vi "BLD_Analysis.vi"() -> ()   [LabVIEW 2019]
uses:
  <vilib>/Analysis/5stat.llb/RMS (DBL).vi
  <vilib>/Analysis/baseanly.llb/Mean (DBL).vi
  <vilib>/express/express analysis/Spectral/Block/exnSpectralBlock spectral measurements power poly.vi
  <vilib>/express/express analysis/Spectral/Block/exnSpectralBlock spectral measurements power DDT.vi
  <vilib>/express/express analysis/Spectral/XNode/ExpressSpectralMeasurementsBlockNode.xnode
  <vilib>/Analysis/NI_AALBase.lvlib
  <vilib>/Analysis/NI_AALPro.lvlib
panel:
  in  "Sensitivity (V)":dbl=100000.0 format="%#_6p"
  in  "Tc (s)":i32=10000 format="%.0p"
  in  "Sampling Rate (Hz)":dbl=100000.0 format="%#_6p"
  in  "Samples (#)":i32=10000 format="%.0p"
  out "data":dynamicdata(graph) caption="APD Output"
  out "Photons/Pulse":ext=-1.22632021926945247725 format="%#.0g"
  in  "Repetition Rate (Hz)":ext[unit]=80000000.0 format="%#_6p"
  in  "Wavelength (m)":dbl=4e-07 format="%#_6p"
  out "Photons/Second":ext[unit]=-98105617.54155619818 format="%#.0p"
  out "Noise (W)":dbl=6.138754193845233e-11 format="%#.2p"
  out "Mean Power (W)":dbl=-4.8720373573303983e-11 format="%#.3p"
  in  "Gain (V/W)":dbl=2500000.0 format="%#_6p"
  in  "stop":bool
  out "Power Spectrum":dynamicdata(graph)=[{"t0"=timestamp(0 s since 1904-01-01), "dt"=1.0000000032596297, "Y"=array[25000 elements], "attributes"=variant("NI_ChannelName"=variant(string "Voltage (Power Spectrum)"), "NI_OriginalChannelName"=variant(string "Voltage"), "NI_UnitDescription"=variant(string "Volts"))}]
  # "Optical Input"
  # "APD"
  # "Lock-in"
  # "DAQ"
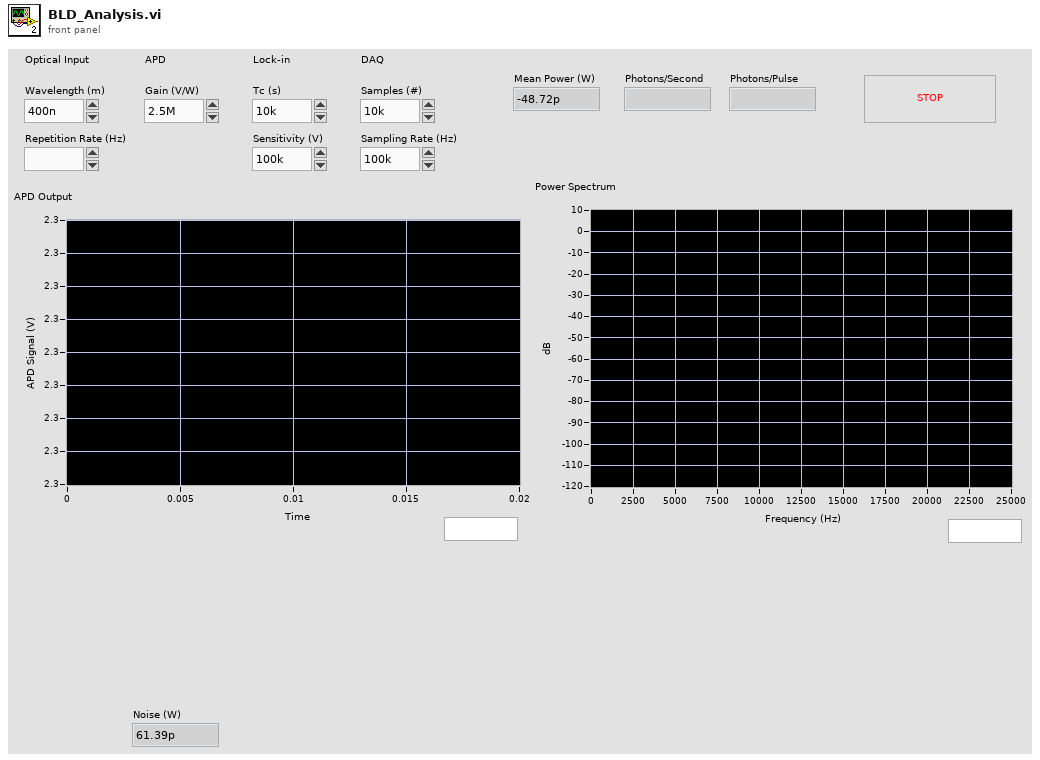
[diagram p1: front panel]
types:
  T1 = cluster{"averaging mode":u16, "weighting mode":u16, "number of averages":u32}
  T2 = cluster{"dB On (F)":bool, "unwrap phase (F)":bool, "convert to degree (F)":bool}
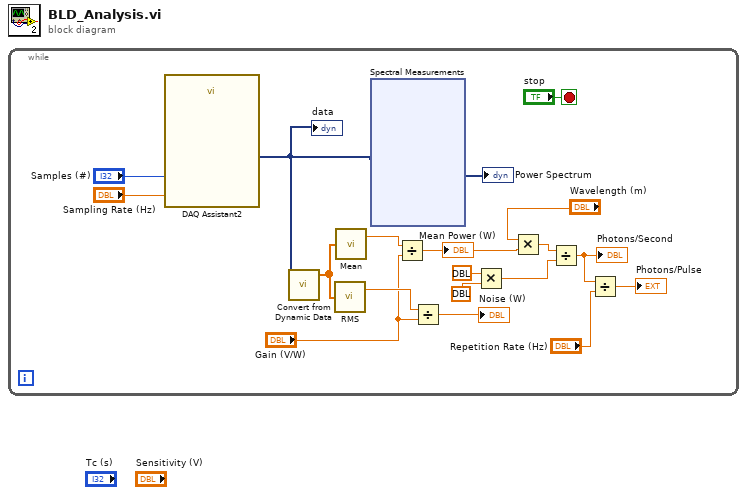
[diagram p0: block diagram]
diagram:
  n1 = while {
    stop <- "stop" stop-if-true
    n2 = call "DAQ Assistant2"("rate"="Sampling Rate (Hz)", "number of samples"="Samples (#)") -> ("data"=w3:dynamicdata)  [unwired: 15 in, 2 out]
    "data" <- w3
    n3 = call "Convert from Dynamic Data"("Dynamic Data Type"=w3) -> ("Array"=w16:dbl[])  [unwired: 3 in]
    n4 = call-poly <vilib>:"RMS.vi"("X"=w16) -> ("rms value"=w15:dbl)  [unwired: 1 out]
    n5 = call-poly <vilib>:"Mean.vi"("X"=w16) -> ("mean"=w17:dbl)  [unwired: 1 out]
    n6 = xnode "Spectral Measurements"("Signals"=w3) -> ("Power Spectrum"=→"Power Spectrum":dynamicdata)  [unwired: 2 in, 2 out]
    n7 = Divide(x=w17, y="Gain (V/W)") -> (x/y=w10:dbl)
    "Mean Power (W)" <- w10
    n8 = Divide(x=w15, y="Gain (V/W)") -> (x/y=→"Noise (W)":dbl)
    n9 = Multiply(x=ext[unit] 6.62607004e-34, y=ext[unit] 299792458.0) -> (x*y=w11:ext[unit])
    n10 = Multiply(x="Wavelength (m)", y=w10) -> (x*y=w9:dbl)
    n11 = Divide(x=w9, y=w11) -> (x/y=w6:ext[unit])
    "Photons/Second" <- w6
    n12 = Divide(x=w6, y="Repetition Rate (Hz)") -> (x/y=→"Photons/Pulse":ext)
  }
